vi "USRP Configure Signal.vi"   [LabVIEW 2016]
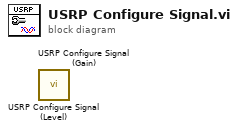
[diagram p0: block diagram]
diagram:
  n1 = call "USRP Configure Signal (Level).vi"() -> ()  [unwired: 9 in, 7 out]
  n2 = call "USRP Configure Signal (Gain).vi"() -> ()  [unwired: 9 in, 7 out]
